vi "Lineup.vi"() -> ()   [LabVIEW 2014]
uses:
  Begin/Global RefNums.vi
  <vilib>/Rock Robotics/WPI/Ultrasonic/WPI_SonarMB1010AnalogRefNum Registry Get.vi
  Begin/Global Variables.vi
  <vilib>/Rock Robotics/WPI/Ultrasonic/WPI_SonarMB1010AnalogGetRange.vi
  <vilib>/addons/control/pid/pid.llb/PID (DBL).vi
  <vilib>/addons/control/pid/NI_PID_pid.lvlib
panel:
  in  "Average Num":dbl=10.0 format="%#_13g"
  in  "Deadband":dbl
  in  "Deadband 2":dbl=0.23 format="%#_13g"
  in  "Angle PID gains 2":T1={"proportional gain (Kc)"=0.15, "integral time (Ti, min)"=0.02, "derivative time (Td, min)"=0.0} {"derivative time (Td, min)" format="%.3f"; "integral time (Ti, min)" format="%.3f"; "proportional gain (Kc)" format="%.3f"}
  in  "Angle output range 2":cluster{"output high":dbl, "output low":dbl}={"output high"=1.0, "output low"=-1.0} {"output low" format="%.2f"; "output high" format="%.2f"}
  in  "Angle Range 2":dbl=0.5 format="%#_13g"
  in  "Forward 2":dbl=15.0 format="%.2f"
  in  "Forward PID gains 2":T1={"proportional gain (Kc)"=0.05, "integral time (Ti, min)"=0.0, "derivative time (Td, min)"=0.0} {"derivative time (Td, min)" format="%.3f"; "integral time (Ti, min)" format="%.3f"; "proportional gain (Kc)" format="%.3f"}
  in  "Forward Output Range 2":cluster{"output high":dbl, "output low":dbl}={"output high"=1.0, "output low"=-1.0} {"output low" format="%.2f"; "output high" format="%.2f"}
  in  "Angle PID gains":T1={"proportional gain (Kc)"=0.09, "integral time (Ti, min)"=0.6, "derivative time (Td, min)"=0.0} {"derivative time (Td, min)" format="%.3f"; "integral time (Ti, min)" format="%.3f"; "proportional gain (Kc)" format="%.3f"}
  in  "Angle output range":cluster{"output high":dbl, "output low":dbl}={"output high"=0.75, "output low"=-0.75} {"output low" format="%.2f"; "output high" format="%.2f"}
  in  "Forward Output Range":cluster{"output high":dbl, "output low":dbl}={"output high"=1.0, "output low"=-1.0} {"output low" format="%.2f"; "output high" format="%.2f"}
  in  "Forward PID gains":T1={"proportional gain (Kc)"=0.05, "integral time (Ti, min)"=0.0, "derivative time (Td, min)"=0.0} {"derivative time (Td, min)" format="%.3f"; "integral time (Ti, min)" format="%.3f"; "proportional gain (Kc)" format="%.3f"}
  in  "Forward Range":dbl=0.3
  in  "Forward":dbl=15.0 format="%.2f"
  in  "Angle Range":dbl=0.5 format="%#_13g"
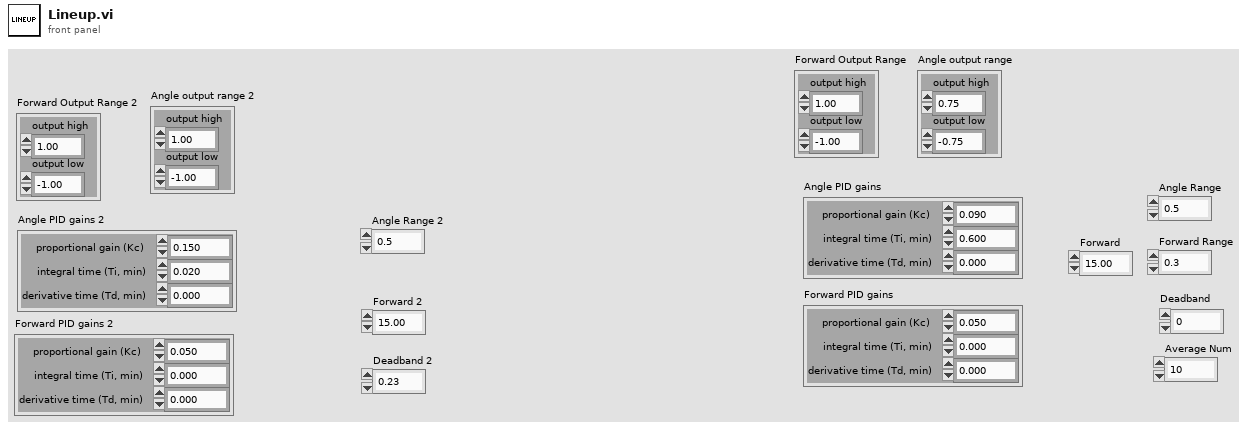
[diagram p1: front panel]
types:
  T1 = cluster{"proportional gain (Kc)":dbl, "integral time (Ti, min)":dbl, "derivative time (Td, min)":dbl}
  T2 = typedef "WPI_SonarMB1010AnalogDeviceRef.ctl" = cluster{"AIDeviceRef":T3, "Scaling factor (V/in)":dbl, "Average Bits":u8}
  T3 = typedef "WPI_AnalogChannelDevRef.ctl" = cluster{"DevStatus":errorcluster, "Controller":T4, "Analog Channel":T5}
  T4 = typedef "FPGA_TypedefAnalogModule.ctl" = enum16{"Controller 1"}
  T5 = typedef "FPGA_AIChannel.ctl" = enum8{"AI 0", "AI 1", "AI 2", "AI 3", "AI MXP 0", "AI MXP 1", "AI MXP 2", "AI MXP 3", "Invalid"}
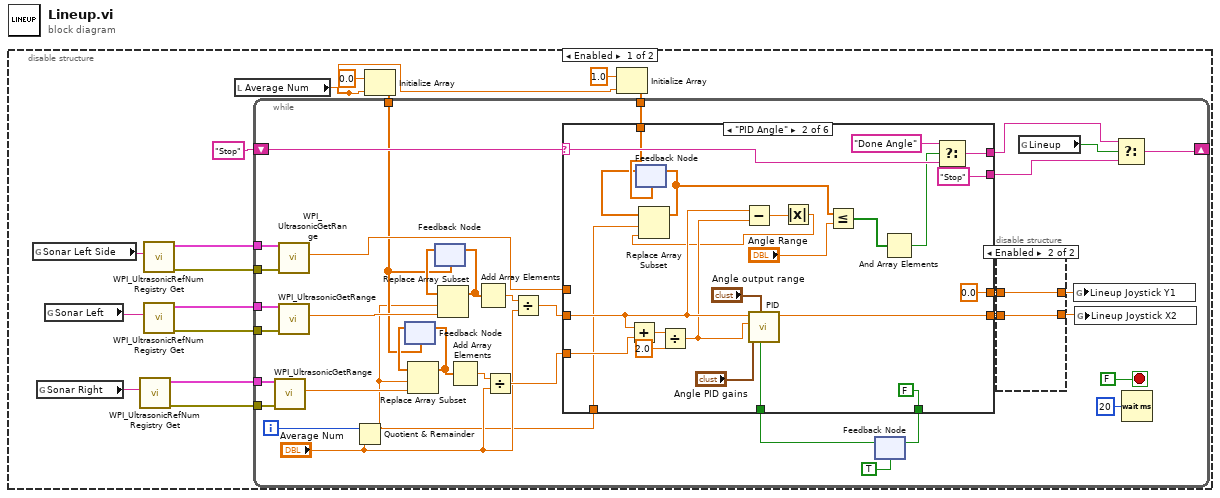
[diagram p0: block diagram]
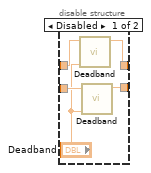
[diagram p2: hidden frame]
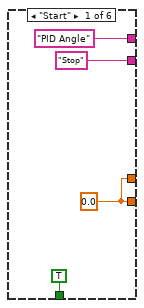
[diagram p3: hidden frame]
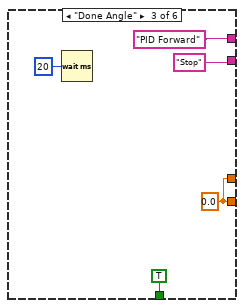
[diagram p4: hidden frame]
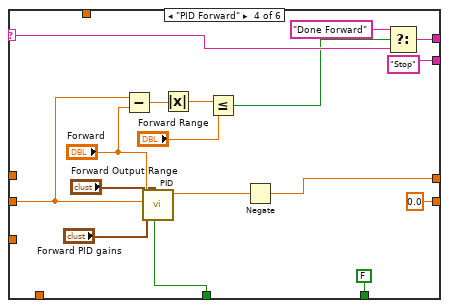
[diagram p5: hidden frame]
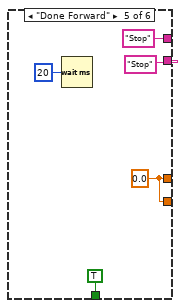
[diagram p6: hidden frame]
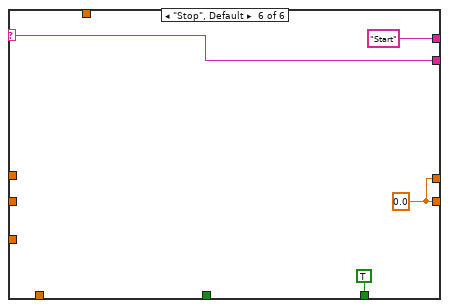
[diagram p7: hidden frame]
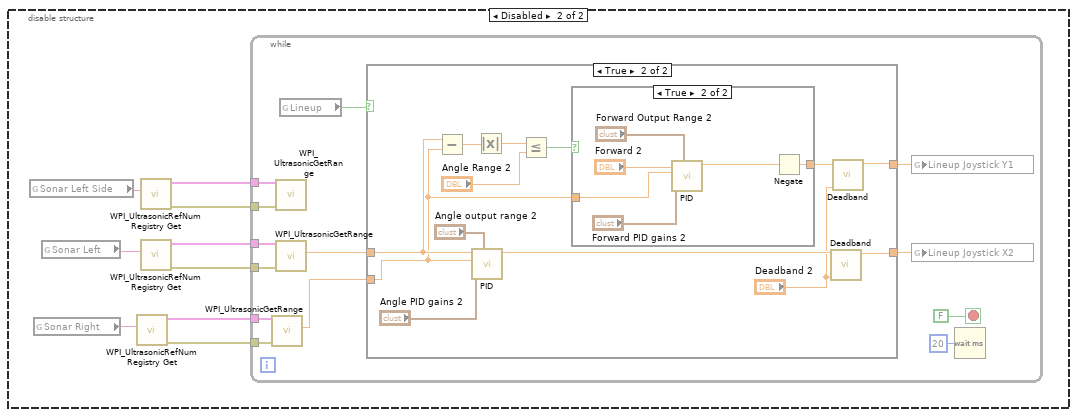
[diagram p8: hidden frame]
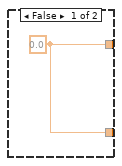
[diagram p9: hidden frame]
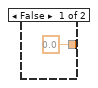
[diagram p10: hidden frame]
diagram:
  n1 = disable-structure shown="Enabled" {
    frame Enabled {
      n2 = global read "Global RefNums.vi" "Sonar Left Side"() -> (w8:string)
      n3 = global read "Global RefNums.vi" "Sonar Right"() -> (w10:string)
      n4 = global read "Global RefNums.vi" "Sonar Left"() -> (w9:string)
      n5 = call-poly <vilib>:"WPI_UltrasonicRefNum Registry Get.vi"("refnum name"=w10) -> ("error out"=w12:errorcluster, "SonarMB1010AnalogDevRef"=w11:T2)  [unwired: 9 in]
      n6 = call-poly <vilib>:"WPI_UltrasonicRefNum Registry Get.vi"("refnum name"=w8) -> ("error out"=w7:errorcluster, "SonarMB1010AnalogDevRef"=w6:T2)  [unwired: 9 in]
      n7 = call-poly <vilib>:"WPI_UltrasonicRefNum Registry Get.vi"("refnum name"=w9) -> ("error out"=w13:errorcluster, "SonarMB1010AnalogDevRef"=w14:T2)  [unwired: 9 in]
      n8 = local read "Average Num"() -> (w1:dbl)
      n9 = Initialize Array(0.0 ("element"), w1) -> (w5:dbl[])
      n10 = Initialize Array(1.0 ("element"), w1) -> (w2:dbl[])
      n11 = while {
        shift-right: [w44] -> _
        shift-left: "Stop" -> [w50]
        tunnel: w14 -> [w49]
        tunnel: w13 -> [w48]
        tunnel: w11 -> [w46]
        tunnel: w12 -> [w47]
        tunnel: w6 -> [w39]
        tunnel: w7 -> [w40]
        tunnel: w5 -> [w22]
        tunnel: w2 -> [w18]
        i -> [w33]
        stop <- FALSE stop-if-true
        n12 = call-poly <vilib>:"WPI_UltrasonicGetRange.vi"("error in"=w47, "SonarMB1010AnalogDevRef"=w46) -> ("Distance"=w24:dbl)  [unwired: 7 in, 2 out]
        n13 = call-poly <vilib>:"WPI_UltrasonicGetRange.vi"("error in"=w40, "SonarMB1010AnalogDevRef"=w39) -> ("Distance"=w38:dbl)  [unwired: 7 in, 2 out]
        n14 = call-poly <vilib>:"WPI_UltrasonicGetRange.vi"("error in"=w48, "SonarMB1010AnalogDevRef"=w49) -> ("Distance"=w23:dbl)  [unwired: 7 in, 2 out]
        n15 = Quotient & Remainder(x=w33, y="Average Num") -> (x-y*floor(x/y)=w16:dbl)  [unwired: 1 out]
        n16 = feedback #1(w22) -> (w26:dbl[])
        n17 = Replace Array Subset(array=w26, new element=w24, index=w16) -> (w27:dbl[])
        n18 = feedback-in #1(w27) -> ()
        n19 = feedback #2(w22) -> (w30:dbl[])
        n20 = Replace Array Subset(array=w30, new element=w23, index=w16) -> (w31:dbl[])
        n21 = feedback-in #2(w31) -> ()
        n22 = Add Array Elements(numeric array=w27) -> (sum=w28:dbl)
        n23 = Add Array Elements(numeric array=w31) -> (sum=w32:dbl)
        n24 = Divide(x=w28, y="Average Num") -> (x/y=w25:dbl)
        n25 = Divide(x=w32, y="Average Num") -> (x/y=w29:dbl)
        n26 = feedback #3(TRUE) -> (w21:bool)
        n27 = case shown="\"PID Angle\"" w50 {
          selector: w50 -> [_ w83 _ w103 _ w116]
          tunnel: ["PID Angle" ("t") w82 "PID Forward" ("t") w102 "Stop" ("t") "Start" ("t")] -> w43
          tunnel: [w62 0.0 ("Lineup Joystick X2") w88 w94 w112 w117] -> w37
          tunnel: [w62 w86 w88 0.0 ("Lineup Joystick X2") w112 w117] -> w35
          tunnel: w29 -> [_ w76 _ w106 _ _]
          tunnel: w25 -> [_ w75 _ _ _ _]
          tunnel: ["Stop" ("t") "Stop" ("t") "Stop" ("t") "Stop" ("t") "Stop" ("t") w116] -> w42
          tunnel: w38 -> [_ _ _ _ _ _]
          tunnel: w21 -> [_ w71 _ w92 _ _]
          tunnel: [TRUE FALSE TRUE FALSE TRUE TRUE] -> w19
          tunnel: w18 -> [_ w69 _ _ _ _]
          tunnel: w16 -> [_ w67 _ _ _ _]
          frame "Start" {
            w62 = 0.0 ("Lineup Joystick X2")
          }
          frame "PID Angle" {
            n28 = Add(x=w76, y=w75) -> (x+y=w74:dbl)
            n29 = feedback #4(w69) -> (w68:dbl[])
            n30 = Divide(x=w74, y=2.0) -> (x/y=w72:dbl)
            n31 = Subtract(x=w76, y=w72) -> (x-y=w85:dbl)
            n32 = call-poly <vilib>:"PID.vi"("reinitialize? (F)"=w71, "output range"="Angle output range", "PID gains"="Angle PID gains", "process variable"=w72, "setpoint"=w76) -> ("output"=w86:dbl)  [unwired: 5 in, 1 out]
            n33 = Absolute Value(x=w85) -> (abs(x)=w66:dbl)
            n34 = Replace Array Subset(array=w68, new element=w66, index=w67) -> (w65:dbl[])
            n35 = feedback-in #4(w65) -> ()
            n36 = Less Or Equal?(x=w65, y="Angle Range") -> (x <= y?=w64:bool[])
            n37 = And Array Elements(Boolean array=w64) -> (logical AND=w63:bool)
            n38 = Select(t="Done Angle", s=w63, f=w83) -> (s? t:f=w82:string)
          }
          frame "Done Angle" {
            w88 = 0.0 ("Lineup Joystick X2")
            n39 = Wait (ms)(milliseconds to wait=u32 20) -> ()  [unwired: 1 out]
          }
          frame "PID Forward" {
            n40 = Subtract(x=w106, y="Forward") -> (x-y=w108:dbl)
            n41 = call-poly <vilib>:"PID.vi"("reinitialize? (F)"=w92, "output range"="Forward Output Range", "PID gains"="Forward PID gains", "process variable"=w106, "setpoint"="Forward") -> ("output"=w95:dbl)  [unwired: 5 in, 1 out]
            n42 = Absolute Value(x=w108) -> (abs(x)=w107:dbl)
            n43 = Less Or Equal?(x=w107, y="Forward Range") -> (x <= y?=w101:bool)
            n44 = Negate(x=w95) -> (-x=w94:dbl)
            n45 = Select(t="Done Forward", s=w101, f=w103) -> (s? t:f=w102:string)
          }
          frame "Done Forward" {
            w112 = 0.0 ("Lineup Joystick X2")
            n46 = Wait (ms)(milliseconds to wait=u32 20) -> ()  [unwired: 1 out]
          }
          frame "Stop", Default {
            w117 = 0.0 ("Lineup Joystick X2")
          }
        }
        n47 = feedback-in #3(w19) -> ()
        n48 = disable-structure shown="Enabled" {
          disable-tunnel: w37 -> [w56 w58]
          disable-tunnel: [w55 w58] -> w36
          disable-tunnel: w35 -> [w54 w57]
          disable-tunnel: [w53 w57] -> w34
          frame Disabled {
            n49 = call "Deadband.vi"("Value to Deadband (default of 0.1)"="Deadband", "Value"=w56) -> ("Deadbanded Value"=w55:dbl)  [unwired: 9 in]
            n50 = call "Deadband.vi"("Value to Deadband (default of 0.1)"="Deadband", "Value"=w54) -> ("Deadbanded Value"=w53:dbl)  [unwired: 9 in]
          }
          frame Enabled {
          }
        }
        n51 = global read "Global Variables.vi" "Lineup"() -> (w41:bool)
        n52 = global write "Global Variables.vi" "Lineup Joystick Y1"(w36) -> ()
        n53 = global write "Global Variables.vi" "Lineup Joystick X2"(w34) -> ()
        n54 = Select(t=w43, s=w41, f=w42) -> (s? t:f=w44:string)
        n55 = Wait (ms)(milliseconds to wait=u32 20) -> ()  [unwired: 1 out]
      }
    }
    frame Disabled {
      n56 = global read "Global RefNums.vi" "Sonar Left Side"() -> (w120:string)
      n57 = global read "Global RefNums.vi" "Sonar Right"() -> (w122:string)
      n58 = global read "Global RefNums.vi" "Sonar Left"() -> (w121:string)
      n59 = call-poly <vilib>:"WPI_UltrasonicRefNum Registry Get.vi"("refnum name"=w122) -> ("error out"=w124:errorcluster, "SonarMB1010AnalogDevRef"=w123:T2)  [unwired: 9 in]
      n60 = call-poly <vilib>:"WPI_UltrasonicRefNum Registry Get.vi"("refnum name"=w120) -> ("error out"=w119:errorcluster, "SonarMB1010AnalogDevRef"=w118:T2)  [unwired: 9 in]
      n61 = call-poly <vilib>:"WPI_UltrasonicRefNum Registry Get.vi"("refnum name"=w121) -> ("error out"=w125:errorcluster, "SonarMB1010AnalogDevRef"=w126:T2)  [unwired: 9 in]
      n62 = while {
        tunnel: w126 -> [w138]
        tunnel: w125 -> [w137]
        tunnel: w123 -> [w135]
        tunnel: w124 -> [w136]
        tunnel: w118 -> [w132]
        tunnel: w119 -> [w133]
        stop <- FALSE stop-if-true
        n63 = call-poly <vilib>:"WPI_UltrasonicGetRange.vi"("error in"=w136, "SonarMB1010AnalogDevRef"=w135) -> ("Distance"=w129:dbl)  [unwired: 7 in, 2 out]
        n64 = call-poly <vilib>:"WPI_UltrasonicGetRange.vi"("error in"=w133, "SonarMB1010AnalogDevRef"=w132) -> ()  [unwired: 7 in, 3 out]
        n65 = call-poly <vilib>:"WPI_UltrasonicGetRange.vi"("error in"=w137, "SonarMB1010AnalogDevRef"=w138) -> ("Distance"=w130:dbl)  [unwired: 7 in, 2 out]
        n66 = global read "Global Variables.vi" "Lineup"() -> (w131:bool)
        n67 = case shown="True" w131 {
          tunnel: w130 -> [_ w147]
          tunnel: w129 -> [_ w146]
          tunnel: [w140 w144] -> w128
          tunnel: [w140 w143] -> w127
          frame False {
            w140 = 0.0
          }
          frame True {
            n68 = Subtract(x=w147, y=w146) -> (x-y=w151:dbl)
            n69 = call-poly <vilib>:"PID.vi"("output range"="Angle output range 2", "PID gains"="Angle PID gains 2", "process variable"=w146, "setpoint"=w147) -> ("output"=w142:dbl)  [unwired: 6 in, 1 out]
            n70 = Absolute Value(x=w151) -> (abs(x)=w150:dbl)
            n71 = Less Or Equal?(x=w150, y="Angle Range 2") -> (x <= y?=w148:bool)
            n72 = case shown="True" w148 {
              tunnel: [0.0 w157] -> w145
              tunnel: w146 -> [_ w155]
              frame False {
              }
              frame True {
                n73 = call-poly <vilib>:"PID.vi"("output range"="Forward Output Range 2", "PID gains"="Forward PID gains 2", "process variable"=w155, "setpoint"="Forward 2") -> ("output"=w158:dbl)  [unwired: 6 in, 1 out]
                n74 = Negate(x=w158) -> (-x=w157:dbl)
              }
            }
            n75 = call "Deadband.vi"("Value to Deadband (default of 0.1)"="Deadband 2", "Value"=w142) -> ("Deadbanded Value"=w143:dbl)  [unwired: 9 in]
            n76 = call "Deadband.vi"("Value to Deadband (default of 0.1)"="Deadband 2", "Value"=w145) -> ("Deadbanded Value"=w144:dbl)  [unwired: 9 in]
          }
        }
        n77 = global write "Global Variables.vi" "Lineup Joystick Y1"(w128) -> ()
        n78 = global write "Global Variables.vi" "Lineup Joystick X2"(w127) -> ()
        n79 = Wait (ms)(milliseconds to wait=u32 20) -> ()  [unwired: 1 out]
      }
    }
  }
